vi "Build Glyph Path.vi"(9 "Version":string, 10 "GlyphLib":string, 11 "VS Public Path":path) -> (3 "Path to Glyph Lib":path)   [LabVIEW 2017, in "Shared Variables CD 2.0 Configuration.lvlib"]
uses:
  Shared Variables CD 2.0/Configuration/Shared Variables CD 2.0 Configuration.lvlib
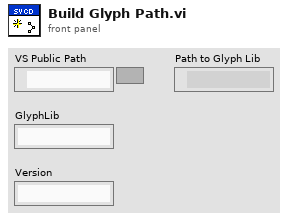
[diagram p1: front panel]
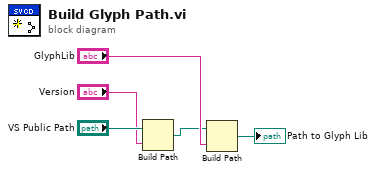
[diagram p0: block diagram]
diagram:
  n1 = Build Path(base path="VS Public Path", name or relative path="Version") -> (appended path=w3:path)
  n2 = Build Path(base path=w3, name or relative path="GlyphLib") -> (appended path=→"Path to Glyph Lib":path)
